vi "UMLEditor_GenerateShortClassIconName.vi"(1 "ClassName":string) -> (0 "ShortClassIconName":string)   [LabVIEW 2012]
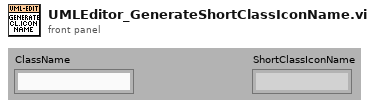
[diagram p1: front panel]
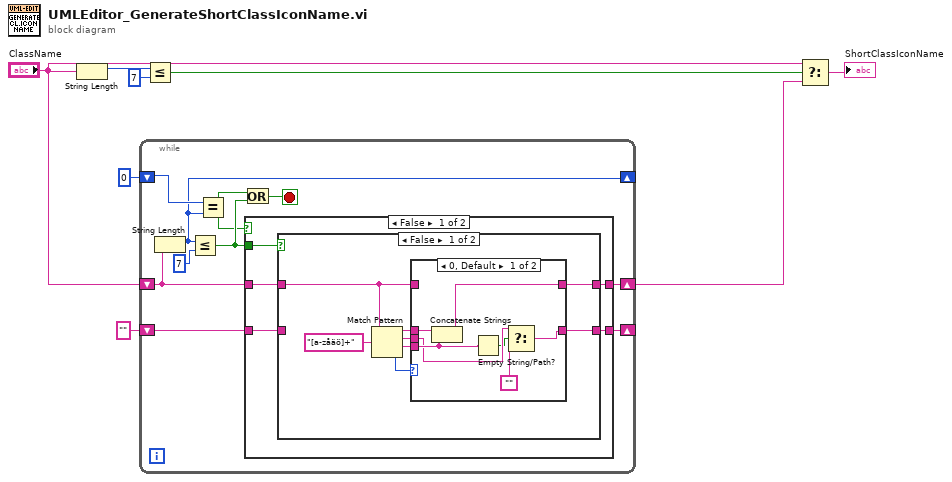
[diagram p0: block diagram]
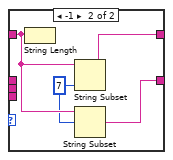
[diagram p2: hidden frame]
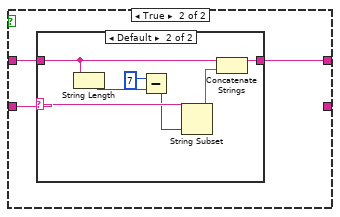
[diagram p3: hidden frame]
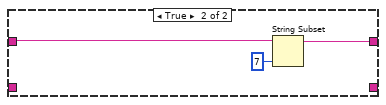
[diagram p5: hidden frame]
diagram:
  n1 = String Length(string="ClassName") -> (length=w8:i32)
  n2 = while {
    shift-right: [w16] -> w4
    shift-left: "ClassName" -> [w17]
    shift-right: [w14] -> _
    shift-left: 0 -> [w15]
    shift-right: [w10] -> _
    shift-left: "" ("ClassName") -> [w9]
    stop <- w11 stop-if-true
    n3 = String Length(string=w17) -> (length=w14:i32)
    n4 = Less Or Equal?(x=w14, y=7) -> (x <= y?=w13:bool)
    n5 = Equal?(x=w15, y=w14) -> (x = y?=w12:bool)
    n6 = Or(x=w12, y=w13) -> (x .or. y?=w11:bool)
    n7 = case shown="False" w12 {
      tunnel: w13 -> [w23 _]
      tunnel: w17 -> [w22 w55]
      tunnel: [w21 w54] -> w16
      tunnel: [w20 _] -> w10
      tunnel: w9 -> [w19 _]
      frame False {
        n8 = case shown="False" w23 {
          tunnel: w22 -> [w26 w44]
          tunnel: [w27 w43] -> w21
          tunnel: [w25 _] -> w20
          tunnel: w19 -> [_ w45]
          frame False {
            n9 = Match Pattern(string=w26, regular expression="[a-zåäö]+") -> (before substring=w30:string, match substring=w24:string, after substring=w29:string, offset past match=w28:i32)  [unwired: 1 out]
            n10 = case shown="0, Default" w28 {
              tunnel: w30 -> [w38 _]
              tunnel: w29 -> [w36 _]
              tunnel: [w37 w42] -> w27
              tunnel: w26 -> [_ w41]
              tunnel: [w34 w39] -> w25
              tunnel: w24 -> [w35 _]
              frame 0, Default {
                n11 = Concatenate Strings(w38, w36) -> (w37:string)
                n12 = Empty String/Path?(string/path=w36) -> (empty?=w32:bool)
                n13 = Select(t=w35, s=w32, f="") -> (s? t:f=w34:string)
              }
              frame -1 {
                w40 = 7 ("length (rest)")
                n14 = String Length(string=w41) -> ()  [unwired: 1 out]
                n15 = String Subset(string=w41, length (rest)=w40) -> (substring=w42:string)  [unwired: 1 out]
                n16 = String Subset(string=w41, offset (0)=w40) -> (substring=w39:string)  [unwired: 1 out]
              }
            }
          }
          frame True {
            n17 = case shown="Default" w45 {
              selector: w45 -> [_ w50]
              tunnel: w44 -> [w46 w53]
              tunnel: [w46 w47] -> w43
              frame "" {
              }
              frame Default {
                n18 = String Length(string=w53) -> (length=w51:i32)
                n19 = Subtract(x=7 ("y"), y=w51) -> (x-y=w49:i32)
                n20 = String Subset(string=w50, length (rest)=w49) -> (substring=w48:string)  [unwired: 1 out]
                n21 = Concatenate Strings(w53, w48) -> (w47:string)
              }
            }
          }
        }
      }
      frame True {
        n22 = String Subset(string=w55, length (rest)=7 ("length (rest)")) -> (substring=w54:string)  [unwired: 1 out]
      }
    }
  }
  n23 = Less Or Equal?(x=w8, y=7) -> (x <= y?=w6:bool)
  n24 = Select(t="ClassName", s=w6, f=w4) -> (s? t:f=→"ShortClassIconName":string)
